vi "Check and Create Kalman Data.vi"(10 "Pk":T1, 11 "x_k":T1) -> (2 "Pk out":T1, 3 "x_k out":T1)   [LabVIEW 2016]
uses:
  <vilib>/Analysis/Matrix/Datatypes/RealMatrix.ctl
  <vilib>/Analysis/Matrix/Numeric/Conversions/Array To Matrix - RA2.vi
  <vilib>/Analysis/7linalg.llb/Create Special Real Matrix.vi
  <vilib>/Analysis/Matrix/NI_Matrix.lvlib
  <vilib>/Analysis/NI_AALPro.lvlib
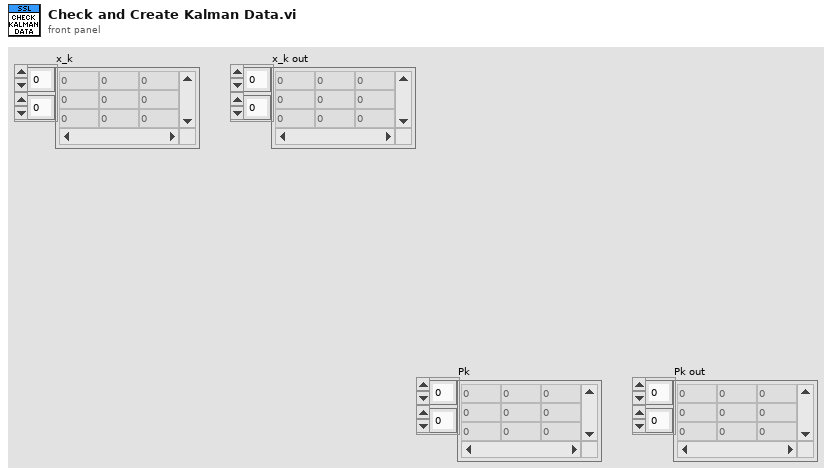
[diagram p1: front panel]
types:
  T1 = typedef "NI_Matrix.lvlib/RealMatrix.ctl" = dbl[][]
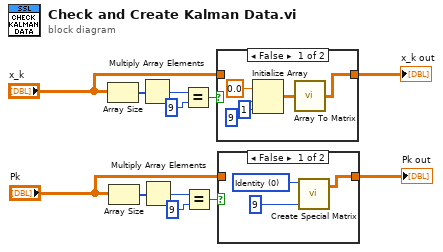
[diagram p0: block diagram]
diagram:
  n1 = Array Size(array="x_k") -> (size(s)=w7:i32[])
  n2 = Array Size(array="Pk") -> (size(s)=w1:i32[])
  n3 = Multiply Array Elements(1:w7) -> (0:w8:i32)
  n4 = Multiply Array Elements(1:w1) -> (0:w2:i32)
  n5 = Equal?(x=w8, y=9) -> (x = y?=w10:bool)
  n6 = Equal?(x=w2, y=9) -> (x = y?=w4:bool)
  n7 = case shown="False" w10 {
    tunnel: "x_k" -> [_ w18]
    tunnel: [w14 w18] -> w12
    frame False {
      n8 = Initialize Array(0.0 ("element"), 9 ("dimension size"), 1 ("dimension size")) -> (w15:dbl[][])
      n9 = call-poly <vilib>:"Array To Matrix.vi"("Real 2D Array"=w15) -> ("Real Matrix"=w14:T1)
    }
    frame True {
    }
  }
  "x_k out" <- w12
  n10 = case shown="False" w4 {
    tunnel: "Pk" -> [_ w22]
    tunnel: [w19 w22] -> w6
    frame False {
      w21 = 0 items=["Identity", "Diagonal", "Toeplitz", "Vandermonde", "Companion", "Hankel", "Hadamard", "Wilkinson", "Hilbert", "Inverse Hilbert", "Rosser", "Pascal"] ("matrix type")
      n11 = call-poly <vilib>:"Create Special Matrix.vi"("matrix type"=w21, "matrix size"=9) -> ("Special Matrix"=w19:T1)  [unwired: 3 in, 1 out]
    }
    frame True {
    }
  }
  "Pk out" <- w6
